vi "Read Build Machine Feed Folderpath.vi"(8 "error in (no error)":errorcluster, 11 "NIPKG_LV in":refnum<class "NIPKG_LV.lvclass">) -> (0 "error out":errorcluster, 2 "Build Machine Feed Folderpath":path, 3 "NIPKG_LV out":refnum<class "NIPKG_LV.lvclass">)   [LabVIEW 2017, in "CL_G3_VIComponentBuilder.lvlib" / "NIPKG_LV.lvclass"]
uses:
  NIPKG_LV.lvclass
  NIPKG_LV.lvclass/NIPKG_LV.ctl
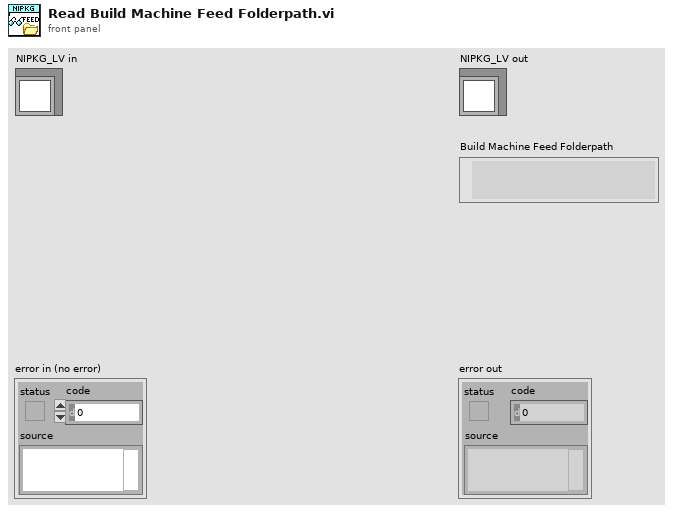
[diagram p1: front panel]
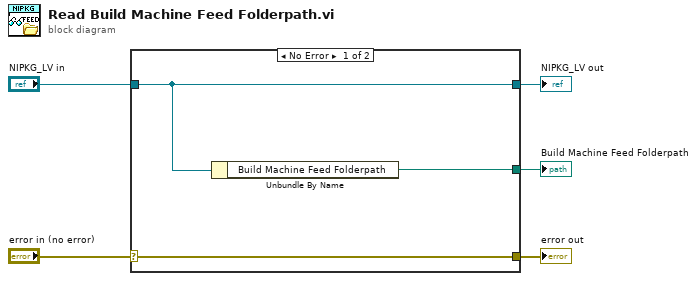
[diagram p0: block diagram]
diagram:
  n1 = case shown="No Error" "error in (no error)" {
    selector: "error in (no error)" -> [w8 w9]
    tunnel: [w8 w9] -> w4
    tunnel: [w7 w10] -> w2
    tunnel: "NIPKG_LV in" -> [w7 w10]
    tunnel: [w6 _] -> w1
    frame No Error {
      n2 = Unbundle By Name(w7) -> ("Build Machine Feed Folderpath"=w6:path)
    }
    frame Error {
    }
  }
  "error out" <- w4
  "NIPKG_LV out" <- w2
  "Build Machine Feed Folderpath" <- w1
